vi "To Variant.vi"(0 "Obj in":refnum<class "Gate.lvclass">, 11 "error in (no error)":errorcluster) -> (4 "Obj out":refnum<class "Gate.lvclass">, 8 "Array":variant[](array[variant]), 15 "error out":errorcluster)   [LabVIEW 2020, in "Gate.lvclass"]
uses:
  Gate.lvclass
  Shape.ctl
  Gate.lvclass/Gate.ctl
  Koop/KObject Class/KObject.lvclass
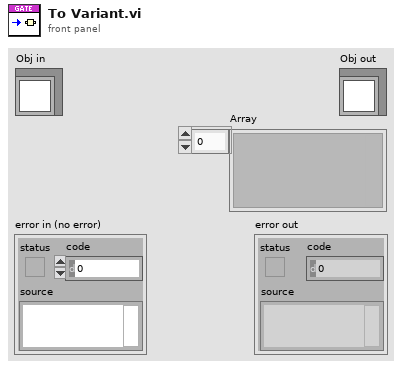
[diagram p1: front panel]
types:
  T1 = typedef "Gate.lvclass/Shape.ctl" = enum16{"OFF", "Rectangle", "Sine-squared", "Trapezoid"}
  T2 = typedef "Gate.lvclass/Serialized.ctl" = cluster{"Shape":T1, "Delay (ms)":dbl, "Duration (ms)":dbl, "Ramp (ms)":dbl, "Repeat":bool, "Rate (Hz)":dbl, "Trepeat (ms)":dbl, "Recycle":bool, "Down (ms)":dbl, "Asymmetric":bool, "Invert":bool, "Delta (dB)":dbl}
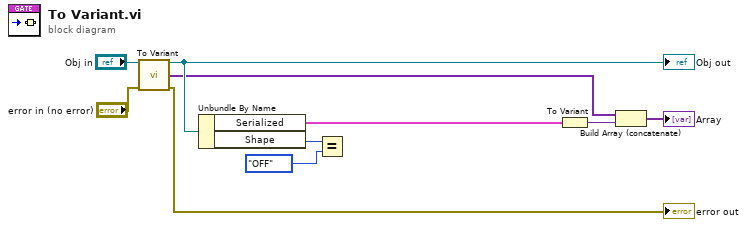
[diagram p0: block diagram]
diagram:
  n1 = call-parent "To Variant.vi"("KObject in"="Obj in", "error in (no error)"="error in (no error)") -> ("KObject out"=w6:refnum<class "Gate.lvclass">, "Array"=w5:variant[], "error out"=→"error out":errorcluster)  [unwired: 11 in]
  "Obj out" <- w6
  n2 = Unbundle By Name(w6) -> ("Serialized"=w1:T2, "Shape"=w3:T1)
  n3 = Equal?(x=w3, y=Shape."OFF") -> ()  [unwired: 1 out]
  n4 = To Variant(anything=w1) -> (Variant=w7:variant)
  n5 = Build Array (concatenate)(w5, w7) -> (→"Array":variant[])
